vi "Create2DArray.vi"(4 "Sequence Context":refnum<k7>) -> (0 "error out":errorcluster)   [LabVIEW 2011]
doc: "Generates a two dimensional array of data and writes it to a TestStand Local Variable using the TestStand API."
uses:
  <vilib>/addons/TestStand/_TSUtility.llb/TestStand API Enumerations.ctl
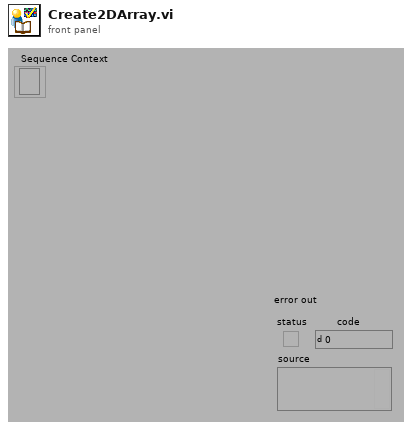
[diagram p1: front panel]
types:
  T1 = typedef "TestStand API Enumerations.ctl" = enum16{"LoadPrototypeOption_NoOptions", "LoadPrototypeOption_MapExistingParameters", "OpenFile_NoOptions", "OpenFile_DisableUseAbsPathCheck", "OpenFile_InitialSetUseAbsPathCheck", "OpenFile_InitialUnsetUseAbsPathCheck", "OpenFile_UseAbsolutePath", "OpenFile_UseRelativePath", "OpenFile_ResolveNonExistentFile", "OpenFile_FileMustNotExist", "OpenFile_SaveAsDialog", "OpenFile_HideUseAbsPathCheck", "OpenFile_ShowBrowseIntoLLBCheck", "OpenFile_SelectDirectoriesOnly", "OpenFile_HideMultiSelectListCtrl", "OpenFile_ModalToAppMainWind", "OpenFile_InitialSetBrowseIntoLLB", "OpenFile_UseSequenceFileFilters", "OpenFile_IgnoreInitialPathExtension", "OpenFile_SubstituteMacrosByDefault", "ExecMask_BreakpointsEnabled", "ExecMask_BreakWhileTerminating", "ExecMask_BreakOnRunTimeError", "ExecMask_TracingEnabled", "ExecMask_TraceIntoSetupCleanup", "ExecMask_TraceIntoPrePostCallbacks", "ExecMask_TraceIntoPostActionCallbacks", "ExecMask_TraceIntoSeparateExecutionCallbacks", "ExecMask_TraceIntoEntryPoints", "ExecMask_TraceIntoSequenceCallsMarkedAsTraceOff", "ExecMask_TraceWhileTerminating", "ExecMask_TraceAllThreads", "ExecMask_InteractiveRecordResults", "ExecMask_InteractiveRunSetupCleanup", "ExecMask_InteractiveEvaluatePreconditions", "ExecMask_DefaultExecutionMask", "ExecMask_AllowBreakWhileInCodeModules", "RWOption_NoOptions", "RWOption_ValuesOnly", "RWOption_EraseExistingObject", "RWOption_EraseAll", "RWOption_DoNotWriteTypes", "PropOption_NoOptions", "PropOption_InsertIfMissing", "PropOption_DeleteIfExists", "PropOption_DoNothingIfExists", "PropOption_SetOnlyIfDoesNotExist", "PropOption_CoerceBadNumbersToZero", "PropOption_CoerceFromNumber", "PropOption_CoerceFromString", "PropOption_CoerceFromBoolean", "PropOption_CoerceFromReference", "PropOption_CoerceToNumber", "PropOption_CoerceToString", "PropOption_CoerceToBoolean", "PropOption_CoerceToReference", "PropOption_Coerce", "PropOption_InsertElement", "PropOption_RemoveElement", "PropOption_OverrideNotDeletable", "PropOption_NotOwning", "PropOption_ReferToAlias", "PropOption_RequireIdenticalStructure", "PropOption_CaseInsensitive", "PropOption_DoNotRecurse", "PropOption_DoNotShareProperties", "PropOption_CopyAllFlags", "PropOption_DoNotAdoptCurrentName", "PropOption_DecimalPoint_UsePeriod", "PropOption_DecimalPoint_UsePreference", "PropOption_DecimalPoint_UseSystemSetting", "PropOption_DecimalPoint_UseComma", "PropFlags_NotEditable", "PropFlags_PassByReference", "PropFlags_Hidden", "PropFlags_HiddenInTypes", "PropFlags_DontTypeCheckParameter", "PropFlags_Propagate", "PropFlags_PermitPropagation", "PropFlags_IsMeasurementValue", "PropFlags_DontCopyToResults", "PropFlags_IsLimit", "PropFlags_IncludeInReport", "PropFlags_CommentNotEditable", "PropFlags_NameNotEditable", "PropFlags_ExcludeFromComparison", "PropFlags_Shared", "PropFlags_SharedAtRunTime", "PropFlags_ExcludeFromCopy", "PropFlags_UnstructuredProperty", "PropFlags_NotDeletable", "PropFlags_IntermediateExprValue", "PropFlags_SerializeAlias", "GetSeqFile_NoOptions", "GetSeqFile_PreloadModules", "GetSeqFile_UpdateFromDisk", "GetSeqFile_AllowTypeConflicts", "GetSeqFile_CheckModelOptions", "GetSeqFile_FindFile", "GetSeqFile_SearchCurrentDir", "GetSeqFile_DoNotRunLoadCallback", "GetSeqFile_OperatorInterfaceFlags", "GetSeqFile_GetFileOnlyIfInCache", "ExecTypeMask_Normal", "ExecTypeMask_InitiallyHidden", "ExecTypeMask_TracingInitiallyOff", "ExecTypeMask_InitiallySuspended", "ExecTypeMask_NotRestartable", "ExecTypeMask_CloseWindowWhenDone", "ExecTypeMask_BreakOnStepFailure", "ExecTypeMask_BreakOnSequenceFailure", "ExecTypeMask_AutoWaitAtEndOfSequence", "ExecTypeMask_UseSTA", "ExecTypeMask_DisplayPreloadProgress", "ExecTypeMask_DiscardArgumentsWhenDone", "SpecMod_NoOptions", "SpecMod_ReadOnly", "SpecMod_NoSyntaxChecking", "SpecMod_AllowPrototypeChanges", "SpecMod_NoParameterLogging", "HierarchicalExecMask_DontRunSetupAndCleanup", "HierarchicalExecMask_RunRemainingSequence", "HierarchicalExecMask_IgnorePreconditions", "RestartOption_NoOptions", "RestartOption_BreakOnEntry", "RestartOption_OverrideNotRestartable", "RestartOption_BreakOnStepFailure", "RestartOption_BreakOnSequenceFailure", "OpenStatus_InWindow", "PropDlgOption_NoOptions", "PropDlgOption_ModalToAppMainWind", "PropDlgOption_ReadOnly", "PropDlgOption_ShowViewContentsButton", "PropDlgOption_DisableAdvancedButton", "PropDlgOption_DisableNumericFormatButton", "PropDlgOutput_AppliedToAllInstances", "PropDlgOutput_AppliedChanges", "PropDlgOutput_ViewContents", "PropDlgOutput_ModifiedObject", "PropDlgOutput_ModifiedFile", "EvalOption_NoOptions", "EvalOption_DoNotAlterValues", "EvalOption_AllowEmptyExpression", "EvalOption_AllowIndexingEmptyArrays", "EvalOption_CreateNonExistentVariables", "EvalOption_ForErrorChecking", "EvalOption_IgnoreNoValidationDirective", "ResetTypeInst_NoOptions", "ResetTypeInst_ResetValues", "ResetTypeInst_ResetFlags", "ResetTypeInst_RecurseSubProperties", "CheckForModifiedTypes_UseStationOptions", "CheckForModifiedTypes_AutoIncrementVersions", "CheckForModifiedTypes_Prompt", "CheckForModifiedTypes_NoAction", "CheckForModifiedTypes_RemoveTypesModifiedMark", "LoadTypePaletteOptions_NoOptions", "LoadTypePaletteOptions_DisplayErrors", "DebugOption_NoOptions", "DebugOption_StackChecking", "DebugOption_BufferChecking", "DebugOption_ReportObjectLeaks", "DebugOption_SendOutputMessagesToDebugger", "DebugOption_ReportKnownOSandComponentProblems", "WinFileDlg_READONLY", "WinFileDlg_OVERWRITEPROMPT", "WinFileDlg_HIDEREADONLY", "WinFileDlg_NOCHANGEDIR", "WinFileDlg_SHOWHELP", "WinFileDlg_ENABLEHOOK", "WinFileDlg_ENABLETEMPLATE", "WinFileDlg_ENABLETEMPLATEHANDLE", "WinFileDlg_NOVALIDATE", "WinFileDlg_ALLOWMULTISELECT", "WinFileDlg_EXTENSIONDIFFERENT", "WinFileDlg_PATHMUSTEXIST", "WinFileDlg_FILEMUSTEXIST", "WinFileDlg_CREATEPROMPT", "WinFileDlg_SHAREAWARE", "WinFileDlg_NOREADONLYRETURN", "WinFileDlg_NOTESTFILECREATE", "WinFileDlg_NONETWORKBUTTON", "WinFileDlg_NOLONGNAMES", "WinFileDlg_EXPLORER", "WinFileDlg_NODEREFERENCELINKS", "WinFileDlg_LONGNAMES", "WinFileDlg_ENABLEINCLUDENOTIFY", "WinFileDlg_ENABLESIZING", "WinFileDlg_DONTADDTORECENT", "WinFileDlg_FORCESHOWHIDDEN", "CommonDlgOption_NoOptions", "CommonDlgOption_ModalToAppMainWind", "CommonDlgOption_ReadOnly", "ArrayBounds_NoOptions", "ArrayBounds_InitializeArray", "ArrayBounds_ReturnOkCancel", "EditPaths_NoOptions", "EditPaths_AllowEditOfReadOnlyFiles", "EditPaths_ModalToAppMainWind", "EditPaths_ReadOnly", "BrowseExpr_NoOptions", "BrowseExpr_UsesCRLF", "BrowseExpr_ModalToAppMainWind", "BrowseExpr_NoContextMenus", "BrowseExpr_ForViewingTypes", "WorkspaceBrowserDlgOption_NoOptions", "WorkspaceBrowserDlgOption_ModalToAppMainWind", "WorkspaceBrowserDlgOption_Editable", "ToolMenuItem_SeparatorBefore", "ToolMenuItem_Enabled", "ToolMenuItem_EditsSelectedFile", "LoadModule_NoOptions", "LoadModule_IgnoreErrors", "LoadModule_LoadModulesInSubSequences", "LoadModule_EvaluateExpressions", "LoadModule_IgnoreSkippedSteps", "LoadModule_ThrowExceptionOnError", "LoadModule_DoNotPromptToFindFile", "LoadModule_DoNotRunLoadCallbacks", "SCCmdOption_NoOptions", "SCCmdOption_DoNotRecurse", "SCCmdOption_SkipPromptDialog", "SCCmdOption_ShowPromptDialog", "SCCmdOption_SkipErrorDialog", "SCStatus_NotInSC", "SCStatus_InSC", "SCStatus_CheckedOut", "SCStatus_CheckedOutOther", "SCStatus_CheckedOutMultiple", "SCStatus_CheckedOutByUser", "SCStatus_Deleted", "SCStatus_OutOfDate", "StepDescOption_NoOptions", "StepDescOption_Long", "StepDescOption_IncludeBreakpoint", "PropTypeFlags_NoFlags", "PropTypeFlags_NoAutoConvertVersions", "PropTypeFlags_DisableEditingInstanceFlags", "PropTypeFlags_PreventEditingType", "PropTypeFlags_NIInstalledType", "PropTypeFlags_IsModifiedType", "SaveAllSeqFiles_NoOptions", "SaveAllSeqFiles_PromptUser", "ReleaseSeqFile_NoOptions", "ReleaseSeqFile_UnloadFileIfModified", "ReleaseSeqFile_DoNotRunUnloadCallback", "ReleaseSeqFile_UnloadFile", "EditNumFormat_NoOptions", "EditNumFormat_AllowDefaultFormat", "EditNumFormat_ModalToAppMainWind", "SearchOptions_MatchCase", "SearchOptions_WholeWordOnly", "SearchOptions_RegExpr", "SearchOptions_IncludeSubsequenceFiles", "SearchFilterOptions_Locals", "SearchFilterOptions_Parameters", "SearchFilterOptions_FileGlobals", "SearchFilterOptions_Steps", "SearchFilterOptions_CustomStepProps", "SearchFilterOptions_BuiltinStepProps", "SearchFilterOptions_ModuleStepProps", "SearchFilterOptions_StepTypes", "SearchFilterOptions_CustomDataTypes", "SearchFilterOptions_StandardDataTypes", "SearchFilterOptions_BuiltinSeqAndSeqFileProps", "SearchFilterOptions_All", "SearchFilterOptions_TypesOnly", "SearchElement_Name", "SearchElement_Comment", "SearchElement_StringValue", "SearchElement_NumericValue", "SearchElement_BooleanValue", "SearchElement_AllValues", "SearchElement_All", "SearchElement_Attributes", "SearchElement_TypeName", "WatchExpressionFilter_NoOptions", "WatchExpressionFilter_IncludeGlobals", "WatchExpressionFilter_FilterByExecution", "WatchExpressionFilter_FilterBySequenceFile", "WatchExpressionFilter_FilterBySequence", "CustomUIMsgOptions_NoOptions", "CustomUIMsgOptions_SuppressIfTraceSent", "CustomUIMsgOptions_AppliesToAllThreads", "XMLOption_NoOptions", "XMLOption_ExcludeComments", "XMLOption_ExcludeFlags", "XMLOption_ExcludeVersionInfo", "XMLOption_ExcludeArrayPrototypes", "XMLOption_ExcludeEmptyObjects", "XMLOption_UseValueFormatIfDefined", "XMLOption_NoIndentation", "XMLOption_NoCRLF", "XMLOption_UseCRLFInsteadOfLF", "XMLOption_ExcludeAliasObjects", "XMLOption_ExcludeAttributes", "TokenizeOption_NoOptions", "TokenizeOption_PreserveComments", "TokenizeOption_RecognizeIncompleteExpression", "TokenizeOption_RecognizeCPPIdentifiers", "EditBreakAndWatch_NoOptions", "EditBreakAndWatch_ReadOnly", "EditBreakAndWatch_ModalToAppMainWind", "EditBreakAndWatch_DisplayBreakpointTab", "EditBreakAndWatch_DisplayWatchExpressionTab", "SaveWorkspaceFile_NoOptions", "SaveWorkspaceFile_PromptUser", "SaveWorkspaceFile_SkipWorkspaceFile", "SaveWorkspaceFile_SkipReadOnlyFiles", "OpenWorkspaceFile_NoOptions", "OpenWorkspaceFile_IgnoreMissingFiles", "OpenWorkspaceFile_SearchCurrentDirectory", "OpenWorkspaceFile_UseSearchDirectories", "BlockFlag_None", "BlockFlag_Open", "BlockFlag_Close", "BlockFlag_Start", "BlockFlag_End", "BlockFlag_Unmatched", "BlockFlag_AppliesToBlockStructure", "ProtectedObjectOption_None", "ProtectedObjectOption_NotEditable", "ProtectedObjectOption_NotViewable", "LockUnlockDialogOption_None", "LockUnlockDialogOption_Lock", "LockUnlockDialogOption_Unlock", "LockUnlockDialogOption_HideRememberPasswordControls", "LockUnlockDialogOption_ModalToAppMainWind", "SequenceFileDifferOptions_NoOptions", "SequenceFileDifferOptions_IgnoreUniqueStepId", "SequenceFileDifferenceType_NoDifference", "SequenceFileDifferenceType_Insert", "SequenceFileDifferenceType_Delete", "SequenceFileDifferenceType_ChangeType", "SequenceFileDifferenceType_ChangeValue", "SequenceFileDifferenceType_ChangeComment", "SequenceFileDifferenceType_ChangeFlags", "SequenceFileDifferenceType_ChangeNumericFormat", "SequenceFileDifferenceType_ArrayDimensions", "SequenceFileDifferenceType_SubProperties", "SequenceFileDifferenceType_UnknownProblem", "SequenceFileDifferenceType_Attributes", "PropValTypeFlag_Any", "PropValTypeFlag_Boolean", "PropValTypeFlag_Number", "PropValTypeFlag_String", "PropValTypeFlag_Reference", "PropValTypeFlag_Container", "PropValTypeFlag_NamedType", "PropValTypeFlag_BooleanArray", "PropValTypeFlag_NumberArray", "PropValTypeFlag_StringArray", "PropValTypeFlag_ReferenceArray", "PropValTypeFlag_ContainerArray", "PropValTypeFlag_ArrayOfNamedType", "PropValTypeFlag_Nothing", "PropValTypeFlag_Object", "PropValTypeFlag_PlainReference", "PropValTypeFlag_PlainContainer", "CreateUndoItemOption_NoOptions", "CreateUndoItemOption_CreateOnly", "SerializationOption_NoOptions", "SerializationOption_UseBinary", "SerializationOption_UseXml", "SerializationOption_SupportNonTypedefMatchingInstances", "NewThreadOption_NoOptions", "NewThreadOption_AutoWaitAtEndOfSequence", "NewThreadOption_InitiallySuspended", "NewThreadOption_UseSTA", "ParseLookupStringOption_NoOptions", "ParseLookupStringOption_TreatArrayIndicesAsSeparateTokens", "GetTemplatesFileOption_NoOptions", "GetTemplatesFileOption_LoadIfNotLoaded", "AcquireLicenseOption_NoOptions", "AcquireLicenseOption_SuppressStartupDialog", "AcquireLicenseOption_SuppressStartupDialogIfAlreadyShown", "AcquireLicenseOption_ShowExitButton", "GotoLocationOption_NoOptions", "GotoLocationOption_DoNotDisplayMessageIfLocationNotFound", "TypeEqualOption_NoOptions", "TypeEqualOption_DoNotCompareDimensions", "TypeEqualOption_DoNotCompareIsObject", "EscapingOption_NoOptions", "EscapingOption_SurroundedByQuotes", "FileModificationIndicatorPolicy_DefaultPolicy", "FileModificationIndicatorPolicy_ExcludeTestStandVersionUpgrade", "VersionConstant_MajorVersion", "VersionConstant_MinorVersion", "VersionConstant_RevisionVersion", "VersionConstant_BuildVersion", "PostResultsCallbackOption_NoOptions", "PostResultsCallbackOption_CallAfterProvisionalResult", "PostResultsCallbackMaskOption_All", "PostResultsCallbackMaskOption_None", "PostResultsCallbackMaskOption_PreStep", "PostResultsCallbackMaskOption_PostStep", "PostResultsCallbackMaskOption_PreInteractive", "PostResultsCallbackMaskOption_PostInteractive", "PostResultsCallbackMaskOption_PostResultListEntry", "PostResultsCallbackMaskOption_PostStepRuntimeError", "PostResultsCallbackMaskOption_PostStepFailure", "PostResultsCallbackMaskOption_PostAction", "PostResultsCallbackMaskOption_SequenceCall", "ReadPropertyObjectFileOption_None", "ReadPropertyObjectFileOption_TypesOnly", "APILocation_ActiveXModule_ActiveXReferenceExpr", "APILocation_ActiveXModule_FilePath", "APILocation_ActiveXModule_RemoteHost", "APILocation_ActiveXParameter_ValueExpr", "APILocation_AdditionalResult_Condition", "APILocation_AdditionalResult_Name", "APILocation_AdditionalResult_ValueToLog", "APILocation_CommonCModule_ModulePath", "APILocation_CommonCModule_ProjectFilePath", "APILocation_CommonCModule_SourceFilePath", "APILocation_CommonCModule_WorkspaceFilePath", "APILocation_CommonCParameter_StringBufferSizeExpr", "APILocation_CommonCParameter_ValueExpr", "APILocation_DllParameter_ImaginaryPartValueExpr", "APILocation_DotNetModule_GetAssembly", "APILocation_DotNetModule_ProjectFilePath", "APILocation_DotNetModule_SolutionFilePath", "APILocation_DotNetModule_SourceFilePath", "APILocation_DotNetParameter_ParameterName", "APILocation_DotNetParameter_ValueExpr", "APILocation_HTBasicModule_SubroutineFilePath", "APILocation_LabVIEWModule_CallName", "APILocation_LabVIEWModule_ClassPath", "APILocation_LabVIEWModule_GetVIAbsolutePath", "APILocation_LabVIEWModule_NodeLibraryName", "APILocation_LabVIEWModule_ProjectPath", "APILocation_LabVIEWModule_RemoteConnectionTimeout", "APILocation_LabVIEWModule_RemoteHost", "APILocation_LabVIEWModule_RemotePortNumber", "APILocation_LabVIEWModule_VIPath", "APILocation_LabVIEWModule_VIType", "APILocation_LabVIEWParameterElement_ElementCaption", "APILocation_LabVIEWParameterElement_ValueExpr", "APILocation_LabVIEWParameter_ParameterCaption", "APILocation_LabVIEWParameter_ValueExpr", "APILocation_None", "APILocation_SequenceCallModule_CustomCPUAffinityForNewThread", "APILocation_SequenceCallModule_NewExecutionBreakOnEntryExpr", "APILocation_SequenceCallModule_NewExecutionModelPath", "APILocation_SequenceCallModule_NewExecutionTypeMaskExpr", "APILocation_SequenceCallModule_RemoteHost", "APILocation_SequenceCallModule_SequenceFilePath", "APILocation_SequenceCallModule_SequenceName", "APILocation_SequenceCallModule_StoreActiveXReferenceExpr", "APILocation_SequenceCallParameter_ValueExpr", "APILocation_SequenceFile_ModelPath", "APILocation_Sequence_DisableResults", "APILocation_StepType_BatchSyncOption", "APILocation_StepType_CustomActionExpression", "APILocation_StepType_CustomFalseAction", "APILocation_StepType_CustomFalseActionTargetByExpr", "APILocation_StepType_CustomTrueAction", "APILocation_StepType_CustomTrueActionTargetByExpr", "APILocation_StepType_DefaultNameExpr", "APILocation_StepType_DescriptionExpr", "APILocation_StepType_EvalPrecondForInteractiveExecution", "APILocation_StepType_FailAction", "APILocation_StepType_FailActionTargetByExpr", "APILocation_StepType_IconName", "APILocation_StepType_IgnoreRTE", "APILocation_StepType_LoopIncExpression", "APILocation_StepType_LoopInitExpression", "APILocation_StepType_LoopStatusExpression", "APILocation_StepType_LoopType", "APILocation_StepType_LoopWhileExpression", "APILocation_StepType_MenuItemNameExpr", "APILocation_StepType_ModuleLoadOption", "APILocation_StepType_ModuleUnloadOption", "APILocation_StepType_MutexNameOrRefExpr", "APILocation_StepType_PassAction", "APILocation_StepType_PassActionTargetByExpr", "APILocation_StepType_PostExpression", "APILocation_StepType_PreExpression", "APILocation_StepType_Precondition", "APILocation_StepType_RecordLoopIterationResults", "APILocation_StepType_RecordResult", "APILocation_StepType_ResultRecordingOption", "APILocation_StepType_RunMode", "APILocation_StepType_StatusExpression", "APILocation_StepType_StepFailCausesSequenceFail", "APILocation_StepType_SwitchExecConnectionLifetime", "APILocation_StepType_SwitchExecEnabled", "APILocation_StepType_SwitchExecMulticonnectMode", "APILocation_StepType_SwitchExecOperation", "APILocation_StepType_SwitchExecOperationOrder", "APILocation_StepType_SwitchExecRoutesToConnect", "APILocation_StepType_SwitchExecRoutesToDisconnect", "APILocation_StepType_SwitchExecVirtualDevice", "APILocation_StepType_SwitchExecWaitForDebounce", "APILocation_StepType_UseMutex", "APILocation_StepType_WindowActivation", "APILocation_Step_BatchSyncOption", "APILocation_Step_CustomActionExpression", "APILocation_Step_CustomFalseAction", "APILocation_Step_CustomFalseActionTargetByExpr", "APILocation_Step_CustomTrueAction", "APILocation_Step_CustomTrueActionTargetByExpr", "APILocation_Step_EvalPrecondForInteractiveExecution", "APILocation_Step_FailAction", "APILocation_Step_FailActionTargetByExpr", "APILocation_Step_IconName", "APILocation_Step_IgnoreRTE", "APILocation_Step_LoopIncExpression", "APILocation_Step_LoopInitExpression", "APILocation_Step_LoopStatusExpression", "APILocation_Step_LoopType", "APILocation_Step_LoopWhileExpression", "APILocation_Step_ModuleLoadOption", "APILocation_Step_ModuleUnloadOption", "APILocation_Step_MutexNameOrRefExpr", "APILocation_Step_PassAction", "APILocation_Step_PassActionTargetByExpr", "APILocation_Step_PostExpression", "APILocation_Step_PreExpression", "APILocation_Step_Precondition", "APILocation_Step_RecordLoopIterationResults", "APILocation_Step_RecordResult", "APILocation_Step_ResultRecordingOption", "APILocation_Step_RunMode", "APILocation_Step_StatusExpression", "APILocation_Step_StepFailCausesSequenceFail", "APILocation_Step_SwitchExecConnectionLifetime", "APILocation_Step_SwitchExecEnabled", "APILocation_Step_SwitchExecMulticonnectMode", "APILocation_Step_SwitchExecOperation", "APILocation_Step_SwitchExecOperationOrder", "APILocation_Step_SwitchExecRoutesToConnect", "APILocation_Step_SwitchExecRoutesToDisconnect", "APILocation_Step_SwitchExecVirtualDevice", "APILocation_Step_SwitchExecWaitForDebounce", "APILocation_Step_UniqueStepId", "APILocation_Step_UseMutex", "APILocation_Step_WindowActivation", "AdditionalResultKind_Call", "AdditionalResultKind_Custom", "AdditionalResultKind_InParameter", "AdditionalResultKind_OutParameter", "AllowAutomaticTypeConflictResolutionOption_Always", "AllowAutomaticTypeConflictResolutionOption_Never", "AllowAutomaticTypeConflictResolutionOption_OnlyIfATypePaletteFileHasTheH", "AllowAutomaticTypeConflictResolutionOption_OnlyIfTypePaletteFilesWillNot", "ApplicationLicense_CustomEditor", "ApplicationLicense_OperatorInterface", "ApplicationLicense_SequenceEditor", "ApplicationLicense_Unspecified", "ApplicationSite_DefaultSite", "ApplicationSite_ItemList", "ApplicationSite_PropertyBrowser", "ApplicationSite_Settings", "ApplicationSite_Variables", "BatchSyncOption_NoSync", "BatchSyncOption_OneThreadOnly", "BatchSyncOption_Parallel", "BatchSyncOption_Serial", "BatchSyncOption_UseModelSetting", "BatchSyncOption_UseSeqFileSetting", "CPUAffinityForNewThreadOption_UseAffinityOfCaller", "CPUAffinityForNewThreadOption_UseAllCPUs", "CPUAffinityForNewThreadOption_UseCustomAffinity", "CPUAffinityForNewThreadOption_UseStationOption", "CallbackType_ModelPostError", "CallbackType_ModelPostFail", "CallbackType_ModelPostInteractive", "CallbackType_ModelPostResult", "CallbackType_ModelPostResults", "CallbackType_ModelPostStep", "CallbackType_ModelPreInteractive", "CallbackType_ModelPreStep", "CallbackType_SeqFilePostError", "CallbackType_SeqFilePostFail", "CallbackType_SeqFilePostInteractive", "CallbackType_SeqFilePostResult", "CallbackType_SeqFilePostResults", "CallbackType_SeqFilePostStep", "CallbackType_SeqFilePreInteractive", "CallbackType_SeqFilePreStep", "CallbackType_StationPostError", "CallbackType_StationPostFail", "CallbackType_StationPostInteractive", "CallbackType_StationPostResult", "CallbackType_StationPostResults", "CallbackType_StationPostStep", "CallbackType_StationPreInteractive", "CallbackType_StationPreStep", "CheckedState_Checked", "CheckedState_Indeterminate", "CheckedState_Unchecked", "CodeTemplateType_CVI", "CodeTemplateType_CppOrC", "CodeTemplateType_HTBasic", "CodeTemplateType_LabVIEW", "CodeTemplateType_Legacy", "CodeTemplateType_VisualBasicDotNet", "CodeTemplateType_VisualCSharpDotNet", "CodeTemplateType_VisualCppDotNet", "ConflictHandler_Error", "ConflictHandler_Prompt", "ConflictHandler_UseGlobalType", "CopyLocationsOption_DeepCopy", "CopyLocationsOption_ShallowCopy", "DecimalPoint_UseComma", "DecimalPoint_UsePeriod", "DecimalPoint_UsePreference", "DecimalPoint_UseSystemSetting", "EditKind_ChangeObject", "EditKind_ChangeRepresentation", "EditKind_ChangeRunMode", "EditKind_ChangeSequenceFileProperties", "EditKind_ChangeSequenceProperties", "EditKind_ChangeStep", "EditKind_ChangeValue", "EditKind_DeleteProperty", "EditKind_DeleteSequence", "EditKind_DeleteStep", "EditKind_InsertProperty", "EditKind_InsertSequence", "EditKind_InsertStep", "EditKind_InsertType", "EditKind_ModifyAttributes", "EditKind_ModifyComment", "EditKind_ModifyFlags", "EditKind_MoveProperty", "EditKind_MoveSequence", "EditKind_MoveStep", "EditKind_MoveType", "EditKind_None", "EditKind_Rename", "EditKind_ReplaceProperty", "Err_AccessDenied", "Err_ActiveXAutomationServerException", "Err_AdapterNoConnectToAutoServer", "Err_AdapterServerConnectionLost", "Err_ArrayIndexOutOfBounds", "Err_ArrayLocked", "Err_AutomationObjNotValid", "Err_BadExpressionError", "Err_BadFileFormat", "Err_BadNetPath", "Err_BadPropertyOrVariableName", "Err_CVIAutoCmdFailed", "Err_CVICantConnectToTecrunServer", "Err_CVIFuncNotFoundInModule", "Err_CVIModuleHasUnresolvedReferences", "Err_CVINotReg", "Err_CVIOleError", "Err_CVIRegGenericReadError", "Err_CVIRegKeyNotFound", "Err_CVIRegValueNotFound", "Err_CVIRegValueTypeMismatch", "Err_CVIUnableToTerminateUserProgInCVI", "Err_CurrentSeqFileNotAvailable", "Err_DDEFail", "Err_DLLNotLoadable", "Err_DiskFull", "Err_DispMissingParamID", "Err_DispMissingParamName", "Err_DispMissingRequiredArg", "Err_DispObsoleteMember", "Err_DispUnknownInterface", "Err_DispUnknownMemberID", "Err_DispUnknownMemberName", "Err_DispUnknownParamID", "Err_DispUnknownParamName", "Err_DispWrongNumPositionalParams", "Err_DoesNotHaveRequiredPrivilege", "Err_DriveNotReady", "Err_DuplicateItemOrValue", "Err_EvaluationContextNotAvailable", "Err_ExprTypeIncompatibleWithParameter", "Err_ExprValueNotSuperSetOfParameter", "Err_FailToRegisterClipFormat", "Err_FileAlreadyExists", "Err_FileFormatIsOutOfDate", "Err_FileFormatNewerThanCurrentVersion", "Err_FileNotConvertableToSeqFile", "Err_FileWasNotFound", "Err_FunctionNotFoundInLib", "Err_IOError", "Err_IllegalOperationOnValue", "Err_IncompatibleParameters", "Err_IndexOutOfRange", "Err_InvalidAdapterName", "Err_InvalidDrive", "Err_InvalidPathname", "Err_ItemCannotBeDeleted", "Err_LVAutoServerError", "Err_LVRTDllNotLoaded", "Err_LVReportedError", "Err_LValueExpected", "Err_MismatchedArrayBounds", "Err_MissingType", "Err_ModuleLoadFailure", "Err_ModuleNotSpecified", "Err_NameAlreadyInUse", "Err_NoError", "Err_NoFileAssoc", "Err_NoItemsInList", "Err_OS_Exception", "Err_ObjectCannotBeAdded", "Err_ObjectTypeIncompatibleWithParameter", "Err_OperationCanceled", "Err_OperationFailed", "Err_OperationInProgress", "Err_OperationOnlyValidWhenSuspended", "Err_OperationTimedOut", "Err_OutOfMemory", "Err_PathNotFound", "Err_ProgramError", "Err_RStringNotFound", "Err_ReadObjectNotFound", "Err_RegistryAccessError", "Err_RegistryItemNotFound", "Err_RemoteHostNotSpecified", "Err_RemoteSequenceError", "Err_RemoteSequenceErrorUnableToConnect", "Err_RemoteSequenceRemoteExecutionDenied", "Err_SequenceAborted", "Err_SequenceTerminated", "Err_SharingViolation", "Err_SingleDimensionalNumericArrayExpected", "Err_SourceCodeControlError", "Err_StackOverflow", "Err_StepTypeNotFound", "Err_ThreadCreationFailed", "Err_TooManyItems", "Err_TypeCannotBeDeleted", "Err_TypeConflict", "Err_TypeLibraryReadError", "Err_TypeMismatchError", "Err_TypeWithDependingInstancesCannotBeDeleted", "Err_UnRecognizedValue", "Err_UnableToAllocateSystemResource", "Err_UnableToCloseFile", "Err_UnableToInitializeOLESystemDLLs", "Err_UnableToLaunchCVI", "Err_UnableToOpenFile", "Err_UnableToPassByReference", "Err_UnexpectedSystemError", "Err_UnexpectedType", "Err_UnknownFunctionOrSequenceName", "Err_UnknownType", "Err_UnknownVariableOrProperty", "Err_ValueIsInvalidOrOutOfRange", "Err_WriteProtected", "Err_WrongNumberOfArrayIndices", "Err_WrongNumberOfParameters", "EvalPrecondOption_EvaluatePrecond", "EvalPrecondOption_NoEvaluatePrecond", "EvalPrecondOption_UseStationOption", "ExecRunState_Paused", "ExecRunState_Running", "ExecRunState_Stopped", "ExecTermState_Aborting", "ExecTermState_KillingThreads", "ExecTermState_Normal", "ExecTermState_Terminating", "ExecTermState_TerminatingInteractive", "FailureAction_GotoCleanup", "FailureAction_None", "FailureAction_UseStationOption", "FileGlobalsScopeOption_AllExecutionsShare", "FileGlobalsScopeOption_SeparateForEachExecution", "FileType_ConfigFile", "FileType_ProjectFile", "FileType_PropertyObjectFile", "FileType_SequenceFile", "FileType_StationGlobalsFile", "FileType_TemplatesFile", "FileType_TypePaletteFile", "FileType_UsersFile", "FileType_WorkspaceFile", "FileVersionInc_Build", "FileVersionInc_Major", "FileVersionInc_Minor", "FileVersionInc_None", "FileVersionInc_Revision", "FileWritingFormat_Binary", "FileWritingFormat_Ini", "FileWritingFormat_Xml", "FindFile_AddDirToSrchList_Ask", "FindFile_AddDirToSrchList_Ask_IgnorePrivileges", "FindFile_AddDirToSrchList_No", "FindFile_AddDirToSrchList_Yes", "FindFile_AddDirToSrchList_Yes_IgnorePrivileges", "FindFile_PromptDisable", "FindFile_PromptEnable", "FindFile_PromptHonorUserPreference", "FindPath_PathIsDir", "FindPath_PathIsFile", "FindPath_PathNotFound", "FindPath_PathNotValid", "InteractiveBranchMode_AllowAll", "InteractiveBranchMode_GotoEnd", "InteractiveBranchMode_Ignore", "InteractiveBranchMode_None", "InteractiveBranchMode_RaiseRTE", "InternalOption_ApplicationManager", "InternalOption_AutomationAdapterUsesDispatchForDualInterfaces", "InternalOption_DisableFloatingWindowsForModalDialogs", "InternalOption_UpdateExternalEnvironments", "InternalOption_WarnOnAPICallThroughDispatchInterface", "LicenseType_BaseDeploymentEngine", "LicenseType_CustomEditorDeployment", "LicenseType_DebugDeploymentEnv", "LicenseType_DevelopmentSystem", "LicenseType_Evaluation", "LicenseType_NoLicense", "LicenseType_OEM", "LicenseType_Other", "LicenseType_Temporary", "LoadOption_DynamicLoad", "LoadOption_PreloadWhenExecuted", "LoadOption_PreloadWhenOpened", "LoadOption_UseStepLoadOption", "LocationKind_Execution", "LocationKind_File", "LocationKind_Type", "ModelOption_NoModel", "ModelOption_RequireSpecificModel", "ModelOption_UseStationModel", "MsgBox_Custom", "MsgBox_Error", "MsgBox_Information", "MsgBox_Warning", "OutputMessageSeverity_Error", "OutputMessageSeverity_Information", "OutputMessageSeverity_Warning", "PerformActionOption_No", "PerformActionOption_Prompt", "PerformActionOption_Yes", "PromptResult_Cancel", "PromptResult_No", "PromptResult_Yes", "PropFlags_NoFlags", "PropValType_Array", "PropValType_Boolean", "PropValType_Container", "PropValType_NamedType", "PropValType_Number", "PropValType_Reference", "PropValType_String", "PropertyObjectElement_Attributes", "PropertyObjectElement_Comment", "PropertyObjectElement_Flags", "PropertyObjectElement_Name", "PropertyObjectElement_None", "PropertyObjectElement_NumericFormat", "PropertyObjectElement_Representation", "PropertyObjectElement_Value", "PropertyRepresentation_Float64", "PropertyRepresentation_Int64", "PropertyRepresentation_None", "PropertyRepresentation_UInt64", "RTEOption_Abort", "RTEOption_Continue", "RTEOption_Ignore", "RTEOption_Retry", "RTEOption_ShowDialog", "ReportConv_FromCRLF", "ReportConv_NoConversion", "ReportConv_ToCRLF", "ResultLogRecordType_BatchDone", "ResultLogRecordType_BatchStart", "ResultLogRecordType_Begin", "ResultLogRecordType_Deleted", "ResultLogRecordType_End", "ResultLogRecordType_NotARecordType", "ResultLogRecordType_OnTheFlyStepResults", "ResultLogRecordType_PostBatch", "ResultLogRecordType_PostUUT", "ResultLogRecordType_PreBatch", "ResultLogRecordType_PreUUT", "ResultLogRecordType_UUTDone", "ResultLogRecordType_UUTStart", "ResultRecordingOption_Disabled", "ResultRecordingOption_Enabled", "ResultRecordingOption_EnabledAndOverrideSequenceSetting", "SCCmd_AddToSC", "SCCmd_CheckIn", "SCCmd_CheckOut", "SCCmd_GetLatest", "SCCmd_RemoveFromSC", "SCCmd_ShowDifferences", "SCCmd_ShowHistory", "SCCmd_ShowProperties", "SCCmd_ShowProviderOptions", "SCCmd_UndoCheckOut", "SearchDirectoryType_AdapterSupportDir", "SearchDirectoryType_ApplicationDir", "SearchDirectoryType_ContainingProjectDir", "SearchDirectoryType_CurrentSequenceFileDir", "SearchDirectoryType_CurrentWorkspaceDir", "SearchDirectoryType_ExplicitDir", "SearchDirectoryType_InitialWorkingDir", "SearchDirectoryType_NIComponentsDir", "SearchDirectoryType_PathEnvironmentVarDir", "SearchDirectoryType_PublicComponentsDir", "SearchDirectoryType_TestStandBinDir", "SearchDirectoryType_TestStandDir", "SearchDirectoryType_TestStandPublicDir", "SearchDirectoryType_UserComponentsDir", "SearchDirectoryType_WindowsDir", "SearchDirectoryType_WindowsSystemDir", "SeqDefValueScope_Execution", "SeqDefValueScope_ExecutionTree", "SeqFileBatchSyncOption_NoSync", "SeqFileBatchSyncOption_OneThreadOnly", "SeqFileBatchSyncOption_Parallel", "SeqFileBatchSyncOption_Serial", "SeqFileBatchSyncOption_UseModelSetting", "SeqFileType_FrontEndCBacks", "SeqFileType_Model", "SeqFileType_Normal", "SeqFileType_StationCBacks", "SeqFileType_Template", "SeqType_Callback", "SeqType_CfgEntryPoint", "SeqType_ExeEntryPoint", "SeqType_Normal", "SeqType_ReservedCallback", "SetTempFileDirectoryOption_Default", "SetTempFileDirectoryOption_NeverOverride", "SpecifyStepsByUniqueIdOption_Ask", "SpecifyStepsByUniqueIdOption_No", "SpecifyStepsByUniqueIdOption_Yes", "StepGroup_Cleanup", "StepGroup_Main", "StepGroup_Setup", "SwitchExecLifetime_Execution", "SwitchExecLifetime_Manual", "SwitchExecLifetime_Sequence", "SwitchExecLifetime_Step", "SwitchExecLifetime_Thread", "SwitchExecMulticonnectMode_Default", "SwitchExecMulticonnectMode_Multiconnect", "SwitchExecMulticonnectMode_None", "SwitchExecOperationOrder_DisconnectAfterConnect", "SwitchExecOperationOrder_DisconnectBeforeConnect", "SwitchExecOperation_Connect", "SwitchExecOperation_ConnectDisconnect", "SwitchExecOperation_Disconnect", "SwitchExecOperation_DisconnectAll", "TS_Err_AccessDenied", "TS_Err_ActiveXAutomationServerException", "TS_Err_AdapterNoConnectToAutoServer", "TS_Err_AdapterServerConnectionLost", "TS_Err_ArrayDimensionExpected", "TS_Err_ArrayDimensionSizeExpected", "TS_Err_ArrayIndexOutOfBounds", "TS_Err_ArrayLocked", "TS_Err_ArrayTypeExpected", "TS_Err_AutomationObjNotValid", "TS_Err_BadExpressionError", "TS_Err_BadFileFormat", "TS_Err_BadNetPath", "TS_Err_BadPropertyOrVariableName", "TS_Err_CVIAutoCmdFailed", "TS_Err_CVICantConnectToTecrunServer", "TS_Err_CVIFuncNotFoundInModule", "TS_Err_CVIModuleHasUnresolvedReferences", "TS_Err_CVINotReg", "TS_Err_CVIOleError", "TS_Err_CVIRegGenericReadError", "TS_Err_CVIRegKeyNotFound", "TS_Err_CVIRegValueNotFound", "TS_Err_CVIRegValueTypeMismatch", "TS_Err_CVIUnableToTerminateUserProgInCVI", "TS_Err_ConvertedErrorCode", "TS_Err_CurrentSeqFileNotAvailable", "TS_Err_DDEFail", "TS_Err_DLLNotLoadable", "TS_Err_DNAssemblyMissing", "TS_Err_DiskFull", "TS_Err_DispMissingParamID", "TS_Err_DispMissingParamName", "TS_Err_DispMissingRequiredArg", "TS_Err_DispObsoleteMember", "TS_Err_DispUnknownInterface", "TS_Err_DispUnknownMemberID", "TS_Err_DispUnknownMemberName", "TS_Err_DispUnknownParamID", "TS_Err_DispUnknownParamName", "TS_Err_DispWrongNumPositionalParams", "TS_Err_DoesNotHaveRequiredPrivilege", "TS_Err_DriveNotReady", "TS_Err_DuplicateItemOrValue", "TS_Err_EmptyExpressionError", "TS_Err_EvaluateFunctionEmptyExpressionError", "TS_Err_EvaluationContextNotAvailable", "TS_Err_ExprTypeIncompatibleWithParameter", "TS_Err_ExprValueNotSuperSetOfParameter", "TS_Err_FailToRegisterClipFormat", "TS_Err_FileAlreadyExists", "TS_Err_FileFormatIsOutOfDate", "TS_Err_FileFormatNewerThanCurrentVersion", "TS_Err_FileNotConvertableToSeqFile", "TS_Err_FileWasNotFound", "TS_Err_FunctionNotFoundInLib", "TS_Err_IOError", "TS_Err_IllegalOperationOnValue", "TS_Err_IncompatibleParameters", "TS_Err_IndexOutOfRange", "TS_Err_InvalidAdapterName", "TS_Err_InvalidDrive", "TS_Err_InvalidPathname", "TS_Err_InvalidPointer", "TS_Err_InvalidRegularExpression", "TS_Err_ItemCannotBeDeleted", "TS_Err_LVAutoServerError", "TS_Err_LVMissingRequiredArg", "TS_Err_LVRTDllNotLoaded", "TS_Err_LVReportedError", "TS_Err_LVRunTimeEngineError", "TS_Err_LVTypeConversionError", "TS_Err_LValueExpected", "TS_Err_LabVIEWTypeNotSupportedInCVI", "TS_Err_MeasStudioInterfaceNotFound", "TS_Err_MemoryChecking", "TS_Err_MethodOrPropertyNotAvailable", "TS_Err_MismatchedArrayBounds", "TS_Err_MismatchedItems", "TS_Err_MissingType", "TS_Err_ModuleLoadFailure", "TS_Err_ModuleNotSpecified", "TS_Err_NameAlreadyInUse", "TS_Err_NoError", "TS_Err_NoFileAssoc", "TS_Err_NoItemsInList", "TS_Err_OS_Exception", "TS_Err_ObjectCannotBeAdded", "TS_Err_ObjectLocked", "TS_Err_ObjectTypeIncompatibleWithParameter", "TS_Err_OperationCanceled", "TS_Err_OperationFailed", "TS_Err_OperationInProgress", "TS_Err_OperationOnlyValidWhenSuspended", "TS_Err_OperationTimedOut", "TS_Err_OutOfMemory", "TS_Err_PathNotFound", "TS_Err_ProgramError", "TS_Err_RStringNotFound", "TS_Err_ReadObjectNotFound", "TS_Err_RegistryAccessError", "TS_Err_RegistryItemNotFound", "TS_Err_RemoteHostNotSpecified", "TS_Err_RemoteSequenceError", "TS_Err_RemoteSequenceErrorUnableToConnect", "TS_Err_RemoteSequenceRemoteExecutionDenied", "TS_Err_SequenceAborted", "TS_Err_SequenceTerminated", "TS_Err_SharingViolation", "TS_Err_SingleDimensionalNumericArrayExpected", "TS_Err_SourceCodeControlError", "TS_Err_StackOverflow", "TS_Err_StepTypeNotFound", "TS_Err_ThreadCreationFailed", "TS_Err_TooManyItems", "TS_Err_TwoDimensionalNumericArrayExpected", "TS_Err_TypeCannotBeDeleted", "TS_Err_TypeConflict", "TS_Err_TypeLibraryReadError", "TS_Err_TypeMismatchError", "TS_Err_TypePaletteFileLoadErrors", "TS_Err_TypeWithDependingInstancesCannotBeDeleted", "TS_Err_UnRecognizedValue", "TS_Err_UnableToAllocateSystemResource", "TS_Err_UnableToCloseFile", "TS_Err_UnableToInitializeOLESystemDLLs", "TS_Err_UnableToLaunchCVI", "TS_Err_UnableToOpenFile", "TS_Err_UnableToPassByReference", "TS_Err_UnexpectedChangeCount", "TS_Err_UnexpectedSystemError", "TS_Err_UnexpectedType", "TS_Err_UnknownFunctionOrSequenceName", "TS_Err_UnknownType", "TS_Err_UnknownVariableOrProperty", "TS_Err_ValueIsInvalidOrOutOfRange", "TS_Err_VisualStudioAutomationError", "TS_Err_WatchExpressionError", "TS_Err_WriteProtected", "TS_Err_WrongNumberOfArrayIndices", "TS_Err_WrongNumberOfParameters", "TS_Err_XMLError", "TestStandPath_Bin", "TestStandPath_CommonAppData", "TestStandPath_Config", "TestStandPath_LocalAppData", "TestStandPath_NIComponents", "TestStandPath_Public", "TestStandPath_PublicComponents", "TestStandPath_Temp", "TestStandPath_TestStand", "ThreadTerminationOption_Never", "ThreadTerminationOption_Normal", "ThreadTerminationOption_Prompt", "TimeLimitAction_Abort", "TimeLimitAction_KillThreads", "TimeLimitAction_Prompt", "TimeLimitAction_Terminate", "TimeLimitOperation_Aborting", "TimeLimitOperation_Executing", "TimeLimitOperation_Terminating", "TimeLimitType_Exiting", "TimeLimitType_NormalExecution", "TokenCode_Assignment", "TokenCode_Bad", "TokenCode_BinaryInteger", "TokenCode_BitwiseAnd", "TokenCode_BitwiseAndAssignment", "TokenCode_BitwiseNot", "TokenCode_BitwiseOr", "TokenCode_BitwiseOrAssignment", "TokenCode_Colon", "TokenCode_Conditional", "TokenCode_Directive", "TokenCode_DivAssignment", "TokenCode_Divide", "TokenCode_DotDot", "TokenCode_Equal", "TokenCode_ExclusiveOr", "TokenCode_ExclusiveOrAssignment", "TokenCode_FieldSpecifier", "TokenCode_GreaterThan", "TokenCode_GreaterThanEqual", "TokenCode_HexInteger", "TokenCode_Identifier", "TokenCode_Integer", "TokenCode_Integer64", "TokenCode_LeftBrace", "TokenCode_LeftBracket", "TokenCode_LeftParenthesis", "TokenCode_LeftShift", "TokenCode_LeftShiftAssignment", "TokenCode_LessThan", "TokenCode_LessThanEqual", "TokenCode_LogicalAnd", "TokenCode_LogicalNot", "TokenCode_LogicalOr", "TokenCode_Minus", "TokenCode_MinusAssignment", "TokenCode_MinusMinus", "TokenCode_ModAssignment", "TokenCode_Modulus", "TokenCode_MultAssignment", "TokenCode_MultiLineComment", "TokenCode_Multiply", "TokenCode_NotAToken", "TokenCode_NotEqual", "TokenCode_OctalInteger", "TokenCode_Plus", "TokenCode_PlusAssignment", "TokenCode_PlusPlus", "TokenCode_Real", "TokenCode_ReferenceFieldSpecifier", "TokenCode_RightBrace", "TokenCode_RightBracket", "TokenCode_RightParenthesis", "TokenCode_RightShift", "TokenCode_RightShiftAssignment", "TokenCode_Separator", "TokenCode_SingleLineComment", "TokenCode_String", "TokenCode_SymbolicConstant", "TokenCode_UnescapedString", "TokenCode_UnsignedInteger64", "TokenCode_UnterminatedMultiLineComment", "TokenCode_UnterminatedString", "ToolMenuType_Command", "ToolMenuType_Sequence", "ToolMenuType_SequenceFile", "ToolMenuType_SubMenu", "TypeCategory_BuiltinDataTypes", "TypeCategory_CustomDataTypes", "TypeCategory_None", "TypeCategory_StepTypes", "TypeVersionInc_Build", "TypeVersionInc_Major", "TypeVersionInc_Minor", "TypeVersionInc_None", "TypeVersionInc_Revision", "UIMsg_AbortingExecution", "UIMsg_BreakOnBreakpoint", "UIMsg_BreakOnRunTimeError", "UIMsg_BreakOnUserRequest", "UIMsg_CascadeWindows", "UIMsg_ClientFileChanged", "UIMsg_CloseWindows", "UIMsg_DisplayReport", "UIMsg_EndExecution", "UIMsg_EndFileExecution", "UIMsg_EndInteractiveExecution", "UIMsg_GotoLocation", "UIMsg_KillingExecutionThreads", "UIMsg_LocalizationSettingChanged", "UIMsg_ModelState_BeginTesting", "UIMsg_ModelState_EnabledStateSet", "UIMsg_ModelState_Identified", "UIMsg_ModelState_Initializing", "UIMsg_ModelState_PostProcessing", "UIMsg_ModelState_PostProcessingComplete", "UIMsg_ModelState_TestingComplete", "UIMsg_ModelState_Waiting", "UIMsg_NonTerminatableThreadsArePreventingTermination", "UIMsg_OpenWindows", "UIMsg_OutputMessages", "UIMsg_ProgressPercent", "UIMsg_ProgressText", "UIMsg_PushUndoItem", "UIMsg_RefreshWindows", "UIMsg_ReportChanged", "UIMsg_ReportCollectionChanged", "UIMsg_ReportLocationChanged", "UIMsg_ResumeFromBreak", "UIMsg_ShutDownCancelled", "UIMsg_ShutDownComplete", "UIMsg_StartExecution", "UIMsg_StartFileExecution", "UIMsg_StartInteractiveExecution", "UIMsg_TerminatingExecution", "UIMsg_TerminatingInteractiveExecution", "UIMsg_TerminationCancelled", "UIMsg_TileWindows", "UIMsg_Trace", "UIMsg_TypePaletteFileListChanged", "UIMsg_UserMessageBase", "UnloadOption_AfterSequenceExecution", "UnloadOption_AfterStepExecution", "UnloadOption_OnPreconditionFailure", "UnloadOption_UseStepUnloadOption", "UnloadOption_WithSequenceFile", "WatchExpressionBreakType_None", "WatchExpressionBreakType_OnChange", "WatchExpressionBreakType_OnExpressionTrue", "WinActOption_ActivateWhenStepCompletes", "WinActOption_IfActiveReactivateWhenStepCompletes", "WinActOption_None", "WorkspaceObjType_Folder", "WorkspaceObjType_OtherFile", "WorkspaceObjType_ProjectFile", "WorkspaceObjType_SequenceFile", "WorkspaceObjType_WorkspaceFile", "WriteFileFormat_Current", "WriteFileFormat_TestStand1", "WriteFileFormat_TestStand2", "WriteFileFormat_TestStand201", "WriteFileFormat_TestStand3", "WriteFileFormat_TestStand31", "WriteFileFormat_TestStand35", "WriteFileFormat_TestStand4", "WriteFileFormat_TestStand41", "WriteFileFormat_TestStand42", "WriteFileFormat_TestStand45", "WriteFileFormat_TestStand50", "WriteFileFormat_TestStand51", "TS_Err_CVINonDllModuleNotSupported", "TS_Err_CVIVersionNotSupported", "TS_Err_ExternalServerUnavailable", "TS_Err_Int32Overflow", "TS_Err_NotSupported", "TS_Err_UInt32Overflow", "TS_Err_UnableToOpenDirectory", "TestStandPath_Temporary", "UIMsg_RuntimeError", "WriteFileFormat_TestStand_14_0"}
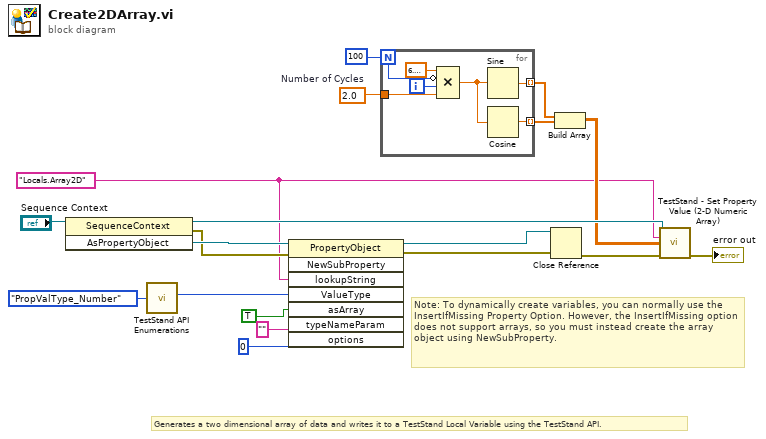
[diagram p0: block diagram]
diagram:
  w8 = 2.0  # Number of Cycles
  w1 = "Locals.Array2D" ("lookupString")
  # "Generates a two dimensional array of data and writes it to a TestStand Local Variable using the TestStand API."
  # "Note: To dynamically create variables, you can normally use the InsertIfMissing Property Option. However, the InsertIfMissing option does not support arrays, so you must instead create the array object using NewSubProperty."
  n1 = invoke class="SequenceContext" method="AsPropertyObject"(reference="Sequence Context") -> (reference out=w10:refnum<k7>, error out=w11:errorcluster, "AsPropertyObject"=w17:refnum<k7>)  [unwired: 2 in]
  n2 = call <vilib>:"TestStand API Enumerations.vi"("Enumeration"=TestStand_API_Enumerations."PropValType_Number") -> ("Value"=w13:i32)  [unwired: 4 out]
  n3 = invoke class="PropertyObject" method="NewSubProperty"(reference=w17, error in=w11, "lookupString"=w1, "ValueType"=w13, "asArray"=TRUE, "typeNameParam"="" ("typeName"), "options"=0) -> (reference out=w2:refnum<k7>, error out=w3:errorcluster)  [unwired: 1 in, 6 out]
  n4 = for {
    N: 100 ("samples") -> [w24]
    tunnel: [w26] -> w5 mode=indexing
    tunnel: w8 -> [w22]
    tunnel: [w20] -> w6 mode=indexing
    i -> [w23]
    n5 = Compound Arithmetic op=MULTIPLY(6.283185307179586, invert w24, w23, w22) -> (w21:dbl)
    n6 = Sine(x=w21) -> (sin(x)=w26:dbl)
    n7 = Cosine(x=w21) -> (cos(x)=w20:dbl)
  }
  n8 = Close Reference(reference=w2, error in (no error)=w3) -> (error out=w9:errorcluster)
  n9 = Build Array(w5, w6) -> (w4:dbl[][])
  n10 = call "TestStand - Set Property Value (2-D Numeric Array).vi"("Sequence Context In"=w10, "Lookup String"=w1, "New Value"=w4, "error in (no error)"=w9) -> ("error out"=→"error out":errorcluster)  [unwired: 1 in, 10 out]
